vi "Flock_CentralException.vi"(8 "Error In":errorcluster) -> (0 "Error Out":errorcluster)   [LabVIEW 2014, in "Flock_ErrorHandling.lvlib"]
doc: "This VI will send the exit command to the Central Process unless an exception for the error has been made within the case structure within the VI. This type of error handling should only be down if it is valid for the Central Process and all local processes because it is a reentrant VI that exists in all processes."
uses:
  Flock_ErrorHandling.lvlib
  CentralProcessMessaging/Flock_Shared_CentralProcessMessaging.lvlib
panel:
  out "resulting string":string
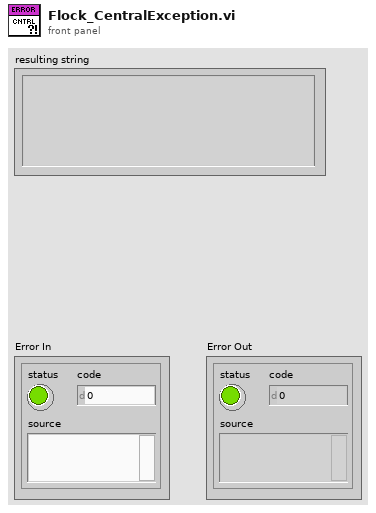
[diagram p1: front panel]
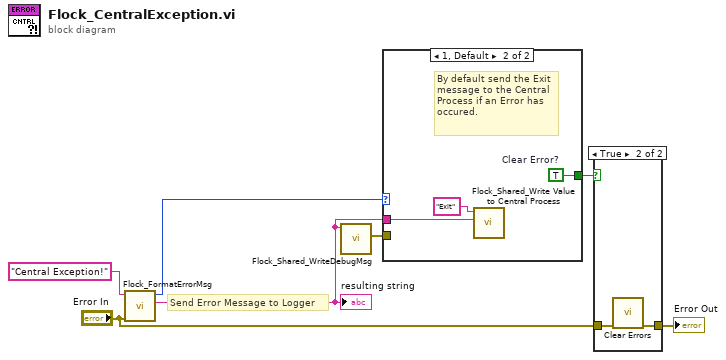
[diagram p0: block diagram]
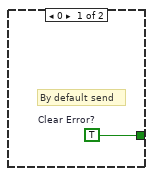
[diagram p3: hidden frame]
diagram:
  # "Send Error Message to Logger"
  n1 = call "Flock_FormatErrorMsg.vi"("error in (no error)"="Error In", "initial string"="Central Exception!") -> ("String"=w6:string, "code"=w5:i32)  [unwired: 8 in]
  "resulting string" <- w6
  n2 = call "Flock_Shared_WriteDebugMsg.vi"("Current Message Case"=w6) -> ("error out"=w1:errorcluster)  [unwired: 10 in]
  n3 = case shown="1, Default" w5 {
    tunnel: w6 -> [_ w10]
    tunnel: [w8 w9] -> w4
    tunnel: w1 -> [_ _]
    frame 0 {
      w8 = TRUE  # Clear Error?
      # "By default send"
    }
    frame 1, Default {
      w9 = TRUE  # Clear Error?
      # "By default send the Exit message to the Central Process if an Error has occured."
      n4 = call "Flock_Shared_Write Value to Central Process.vi"("Message Value"=w10, "Message Name"="Exit") -> ()  [unwired: 9 in, 1 out]
    }
  }
  n5 = case shown="True" w4 {
    tunnel: "Error In" -> [w12 w14]
    tunnel: [w12 w13] -> w2
    frame False {
    }
    frame True {
      n6 = call <vilib>:"Clear Errors.vi"("error in (no error)"=w14) -> ("error out"=w13:errorcluster)  [unwired: 5 in, 1 out]
    }
  }
  "Error Out" <- w2
